vi "Test CI Mediator.vi"() -> ()   [LabVIEW 2014]
uses:
  Core/LabVIEW CI Service/Controls/Job Results - STYP.ctl
  Core/LabVIEW CI Service/Actors/CI Mediator/CI Mediator/CI Mediator.lvclass
  <vilib>/ActorFramework/Message Enqueuer/Message Enqueuer.lvclass/Message Enqueuer.ctl
  Dummy Job/Dummy Job.lvclass
  Core/LabVIEW CI Service/Actors/CI Mediator/CI Mediator Messages/Launch Job Msg/Launch Job Msg.lvclass/Launch Job Msg.ctl
  Core/LabVIEW CI Service/Extensions/LabVIEW Build/LabVIEW Build/LabVIEW Build - STYP.ctl
  <vilib>/ActorFramework/Message Enqueuer/Enqueue.vi
  <vilib>/ActorFramework/Message Priority Queue/Priority Enqueue.vi
  <vilib>/ActorFramework/Stop Msg/Stop Msg.lvclass
  Core/LabVIEW CI Service/Actors/CI Mediator/CI Mediator Messages/Launch Job Msg/Launch Job Msg.lvclass
  <vilib>/ActorFramework/Actor/Actor.lvclass
panel:
  in  "LabVIEW Build":T1={"Executor_Number"="0", "Workspace_Path"=path "P:/alsmith/Sales/users/ACS/LabVIEW Continuous Integration/Workspace", "Build_Spec"="Cooler Executable", "Project_Path"=path "P:/alsmith/Sales/users/ACS/LabVIEW Continuous Integration/Test Project/Complete Solution - Cooler.lvproj", "Auto_Version_Increment"=FALSE}
  in  "LabVIEW Build":bool
  out "Result":T2 {"Status" items=["Service Error"=504, "Abort"=503, "Fail"=500, "Pass"=200]}
  in  "Dummy Job":bool
  in  "stop":bool
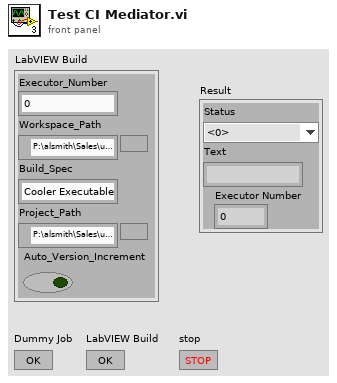
[diagram p1: front panel]
types:
  T1 = cluster{"Executor_Number":string, "Workspace_Path":path, "Build_Spec":string, "Project_Path":path, "Auto_Version_Increment":bool}
  T2 = typedef "Job Results - STYP.ctl" = cluster{"Status":u16, "Text":string, "Executor Number":i32}
  T3 = typedef "LabVIEW Build - STYP.ctl" = cluster{"Executor_Number":string, "Workspace_Path":string, "Build_Spec":string, "Target":string, "Project_Path":string, "Auto_Version_Increment":bool}
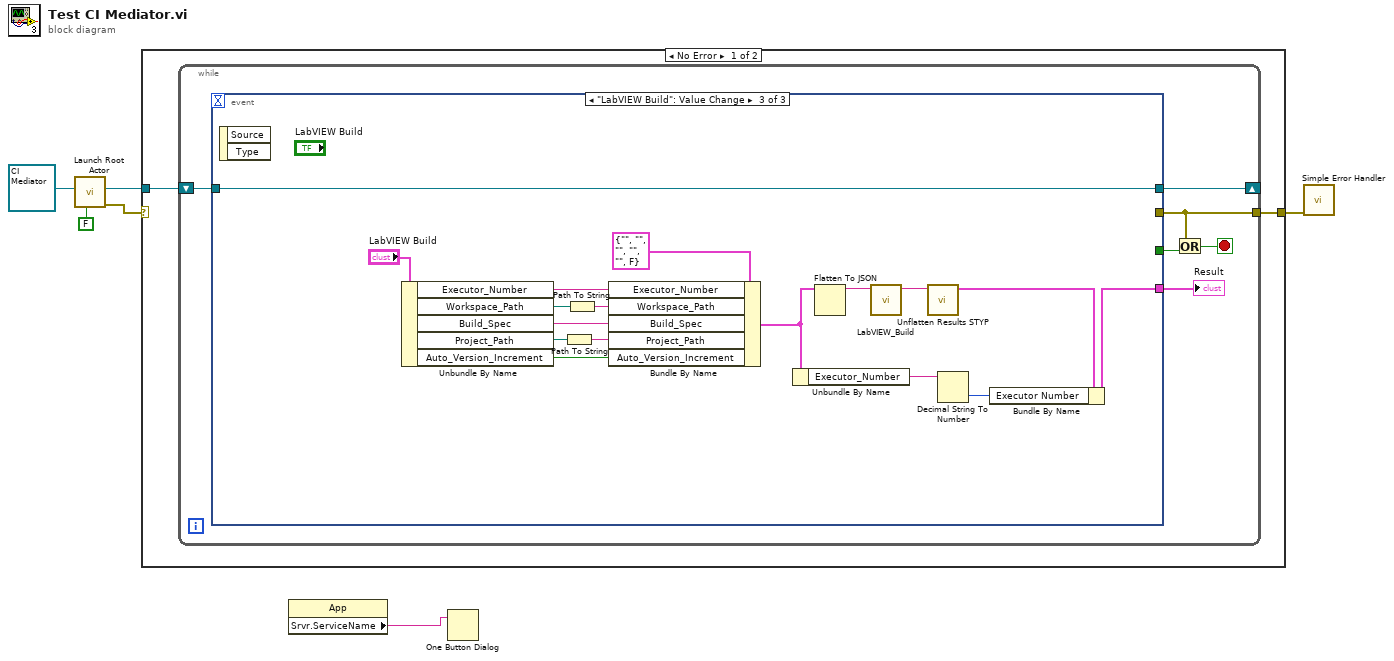
[diagram p0: block diagram]
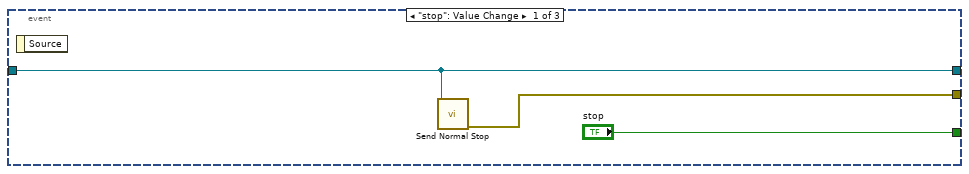
[diagram p2: hidden frame]
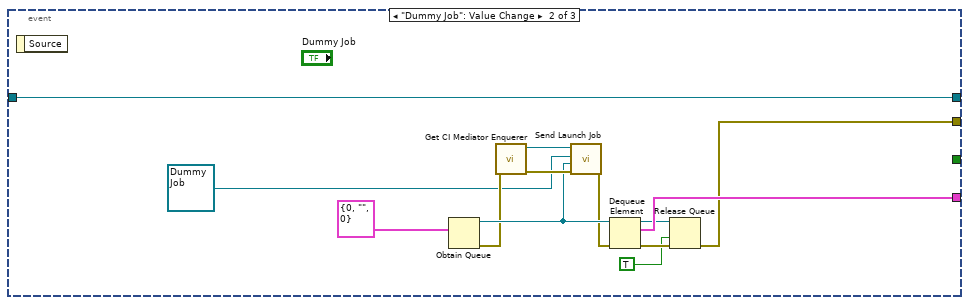
[diagram p3: hidden frame]
diagram:
  n1 = call <vilib>:"Launch Root Actor.vi"("Open Actor Core front panel? (F)"=FALSE, "Actor"=refnum<class "CI Mediator.lvclass"> refnum ("CI Mediator.lvlib:CI Mediator.lvclass")) -> ("error out"=w2:errorcluster, "Actor's Enqueuer"=w3:refnum<class "Message Enqueuer.lvclass">)  [unwired: 8 in]
  n2 = case shown="No Error" w2 {
    selector: w2 -> [_ w48]
    tunnel: [w8 w48] -> w6
    tunnel: w3 -> [w7 _]
    frame No Error {
      n3 = while {
        shift-right: [w13] -> _
        shift-left: w7 -> [w14]
        tunnel: [w12] -> w8
        stop <- w11 stop-if-true
        n4 = event shown="[2] \"LabVIEW Build\": Value Change" {
          selector: _ -> [_ _ _]
          dyn-events: _ -> [_ _ _]
          timeout: _ -> [_ _ _]
          tunnel: w14 -> [w16 w24 w47]
          tunnel: [w16 w24 w47] -> w13
          tunnel: [w15 w20 _] -> w12
          tunnel: ["stop" _ _] -> w10
          tunnel: [_ w21 w32] -> w9
          event "stop": Value Change {
            n5 = event-data() -> ()  [unwired: 1 in, 1 out]
            n6 = call <vilib>:"Send Normal Stop.vi"("Message Enqueuer"=w16) -> ("error out"=w15:errorcluster)  [unwired: 10 in]
          }
          event "Dummy Job": Value Change {
            n7 = event-data() -> ()  [unwired: 1 in, 1 out]
            n8 = Obtain Queue(element data type=T2 {"Status"=0, "Text"="", "Executor Number"=0} ("element")) -> (queue out=w27:refnum<queue>, error out=w26:errorcluster)  [unwired: 4 in, 1 out]
            n9 = call "Get CI Mediator Enquerer.vi"("error in (no error)"=w26) -> ("error out"=w28:errorcluster, "Enquerer"=w30:refnum<class "Message Enqueuer.lvclass">)  [unwired: 9 in]
            n10 = call "Send Launch Job.vi"("error in (no error)"=w28, "Reply Queue"=w27, "Job.lvclass"=refnum<class "Dummy Job.lvclass"> refnum ("Dummy Job.lvclass"), "Message Enqueuer"=w30) -> ("error out"=w25:errorcluster)  [unwired: 6 in, 1 out]
            n11 = Dequeue Element(queue=w27, error in (no error)=w25) -> (queue out=w19:refnum<queue>, element=w21:T2, error out=w22:errorcluster)  [unwired: 1 in, 1 out]
            n12 = Release Queue(queue=w19, force destroy? (F)=TRUE, error in (no error)=w22) -> (error out=w20:errorcluster)  [unwired: 2 out]
          }
          event "LabVIEW Build": Value Change {
            n13 = event-data() -> ()  [unwired: 1 in, 2 out]
            n14 = Unbundle By Name("LabVIEW Build") -> ("Executor_Number"=w43:string, "Workspace_Path"=w38:path, "Build_Spec"=w41:string, "Project_Path"=w36:path, "Auto_Version_Increment"=w42:bool)
            n15 = Path To String(path=w36) -> (string=w35:string)
            n16 = Path To String(path=w38) -> (string=w37:string)
            n17 = Bundle By Name(cluster=T3 {"Executor_Number"="", "Workspace_Path"="", "Build_Spec"="", "Target"="", "Project_Path"="", "Auto_Version_Increment"=FALSE} ("LabVIEW Build"), "Executor_Number"=w43, "Workspace_Path"=w37, "Build_Spec"=w41, "Project_Path"=w35, "Auto_Version_Increment"=w42) -> (w40:T3)
            n18 = Unbundle By Name(w40) -> ("Executor_Number"=w45:string)
            n19 = Flatten To JSON(anything=w40) -> (JSON string=w46:string)  [unwired: 2 in, 1 out]
            n20 = call "LabVIEW_Build.vi"("JSON"=w46) -> ("Result"=w34:string)  [unwired: 10 in]
            n21 = call "Unflatten Results STYP.vi"("Result in"=w34) -> ("Result out"=w33:T2)  [unwired: 10 in]
            n22 = Decimal String To Number(string=w45) -> (number=w31:i32)  [unwired: 2 in, 1 out]
            n23 = Bundle By Name(cluster=w33, "Executor Number"=w31) -> (w32:T2)
          }
        }
        "Result" <- w9
        n24 = Or(x=w12, y=w10) -> (x .or. y?=w11:bool)
      }
    }
    frame Error {
    }
  }
  n25 = property class="App"() -> ("Srvr.ServiceName"=w1:string)  [unwired: 2 in, 2 out]
  n26 = One Button Dialog(message=w1) -> ()  [unwired: 1 in, 1 out]
  n27 = call <vilib>:"Simple Error Handler.vi"("error in (no error)"=w6) -> ()  [unwired: 4 in, 5 out]
